vi "簇转文本处理.vi"(11 "data":variant[](array[variant])) -> (3 "output":string)   [LabVIEW 2016]
uses:
  <vilib>/addons/database/Auxilliary.llb/DB Tools DataTypes.ctl
  <vilib>/addons/database/NI_Database_API.lvlib
  <vilib>/Utility/VariantDataType/VariantType.lvlib
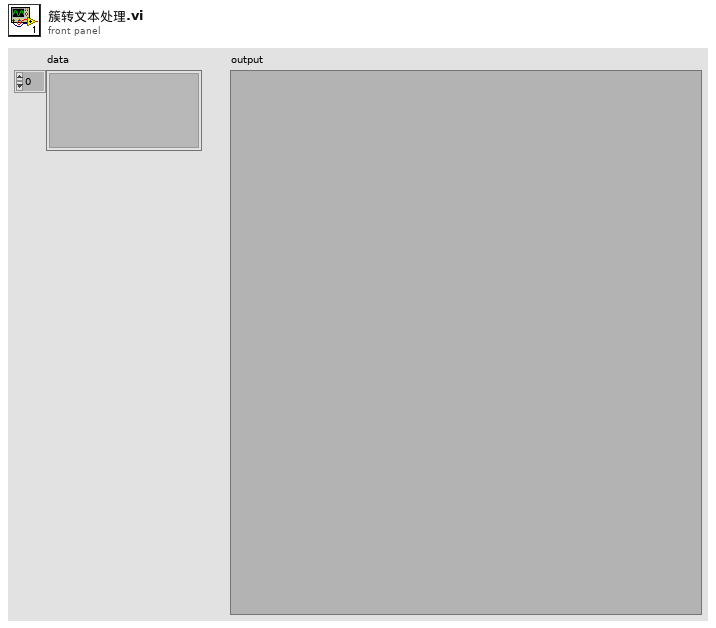
[diagram p1: front panel]
types:
  T1 = typedef "NI_Database_API.lvlib/DB Tools DataTypes.ctl" = enum16{"String", "Long (I32)", "Single (SGL)", "Double (DBL)", "Date/Time", "Binary"}
  T2 = typedef "VariantType.lvlib/Type.ctl" = enum8{"Invalid Type", "Void", "I8", "I16", "I32", "I64", "U8", "U16", "U32", "U64", "Single Float", "Double Float", "Extended Float", "Single Complex", "Double Complex", "Extended Complex", "Enum U8", "Enum U16", "Enum U32", "Enum U64", "Single Float With Unit", "Double Float With Unit", "Extended Float With Unit", "Single Complex with Unit", "Double Complex with Unit", "Extended Complex with Unit", "Boolean", "String", "Path", "Picture", "Tag", "Array", "Cluster", "Variant", "LV Variant", "Waveform", "Timestamp", "Digital Waveform", "Digital Data", "ExpressData", "Refnum", "External Data", "VI", "Poly VI", "LabVIEW Class Instance", "Fixed Point"}
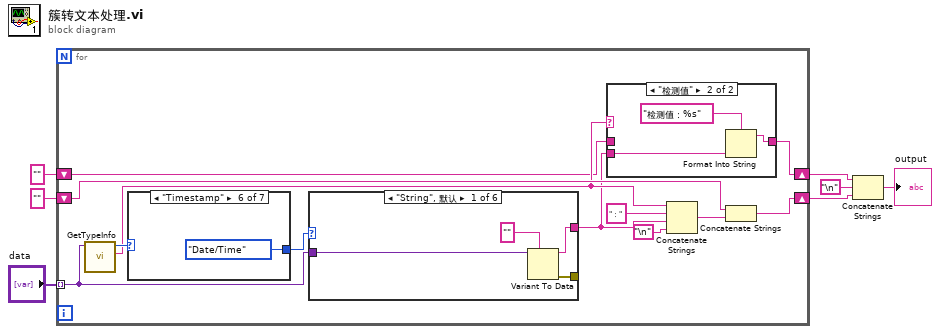
[diagram p0: block diagram]
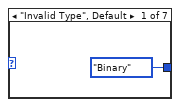
[diagram p3: hidden frame]
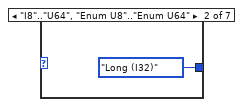
[diagram p4: hidden frame]
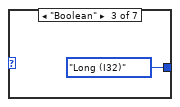
[diagram p5: hidden frame]
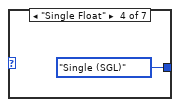
[diagram p6: hidden frame]
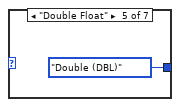
[diagram p7: hidden frame]
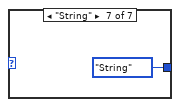
[diagram p8: hidden frame]
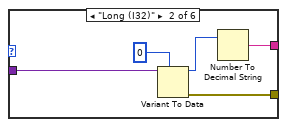
[diagram p9: hidden frame]
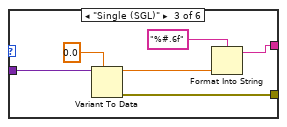
[diagram p10: hidden frame]
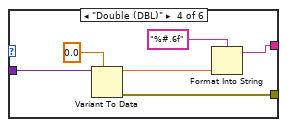
[diagram p11: hidden frame]
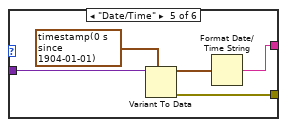
[diagram p12: hidden frame]
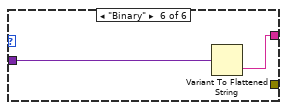
[diagram p13: hidden frame]
diagram:
  n1 = for {
    shift-right: [w15] -> w2
    shift-left: "" -> [w17]
    tunnel: "data" -> [w13] mode=indexing
    shift-right: [w9] -> w4
    shift-left: "" -> [w8]
    n2 = call <vilib>:"GetTypeInfo.vi"("Variant"=w13) -> ("Name"=w11:string, "Type Enum"=w14:T2)  [unwired: 6 in, 3 out]
    n3 = case shown="\"Timestamp\"" w14 {
      tunnel: [DB_Tools_DataTypes."Binary" ("data type") DB_Tools_DataTypes."Long (I32)" ("data type") DB_Tools_DataTypes."Long (I32)" ("data type") DB_Tools_DataTypes."Single (SGL)" ("data type") DB_Tools_DataTypes."Double (DBL)" ("data type") DB_Tools_DataTypes."Date/Time" ("data type") DB_Tools_DataTypes."String" ("data type")] -> w12
      frame "Invalid Type", Default {
      }
      frame "I8".."U64", "Enum U8".."Enum U64" {
      }
      frame "Boolean" {
      }
      frame "Single Float" {
      }
      frame "Double Float" {
      }
      frame "Timestamp" {
      }
      frame "String" {
      }
    }
    n4 = case shown="\"String\", 默认" w12 {
      tunnel: w13 -> [w33 w39 w44 w50 w56 w58]
      tunnel: [w31 w35 w43 w49 w54 _] -> _
      tunnel: [w32 w36 w40 w47 w52 w57] -> w10
      frame "String", Default {
        n5 = Variant To Data(type="", Variant=w33) -> (data=w32:string, error out=w31:errorcluster)  [unwired: 1 in]
      }
      frame "Long (I32)" {
        n6 = Variant To Data(type=0, Variant=w39) -> (data=w37:i32, error out=w35:errorcluster)  [unwired: 1 in]
        n7 = Number To Decimal String(number=w37) -> (decimal integer string=w36:string)  [unwired: 1 in]
      }
      frame "Single (SGL)" {
        n8 = Variant To Data(type=sgl 0.0, Variant=w44) -> (data=w42:sgl, error out=w43:errorcluster)  [unwired: 1 in]
        n9 = Format Into String(format string="%#.6f" ("格式字符串"), w42) -> (resulting string=w40:string)  [unwired: 2 in, 1 out]
      }
      frame "Double (DBL)" {
        n10 = Variant To Data(type=0.0, Variant=w50) -> (data=w48:dbl, error out=w49:errorcluster)  [unwired: 1 in]
        n11 = Format Into String(format string="%#.6f" ("格式字符串"), w48) -> (resulting string=w47:string)  [unwired: 2 in, 1 out]
      }
      frame "Date/Time" {
        n12 = Variant To Data(type=timestamp(0 s since 1904-01-01) ("时间标识"), Variant=w56) -> (data=w53:timestamp, error out=w54:errorcluster)  [unwired: 1 in]
        n13 = Format Date/Time String(seconds (now)=w53) -> (date/time string=w52:string)  [unwired: 2 in]
      }
      frame "Binary" {
        n14 = Variant To Flattened String(Variant=w58) -> (data string=w57:string)  [unwired: 1 out]
      }
    }
    n15 = case shown="\"检测值\"" w11 {
      tunnel: w10 -> [_ w22]
      tunnel: [w20 w21] -> w9
      tunnel: w8 -> [w20 _]
      frame Default {
      }
      frame "检测值" {
        n16 = Format Into String(format string="检测值：%s" ("格式字符串"), w22) -> (resulting string=w21:string)  [unwired: 2 in, 1 out]
      }
    }
    n17 = Concatenate Strings(w11, "：" ("字符串"), w10, "\n") -> (w16:string)
    n18 = Concatenate Strings(w17, w16) -> (w15:string)
  }
  n19 = Concatenate Strings(w4, "\n", w2) -> (→"output":string)
